vi "Background UI Trigger Timer.vi"(8 "error in (no error)":errorcluster, 10 "Backstage Update Peroid (ms)":i32=-1, 11 "VI Ref (calling VI)":refnum<vi>) -> (0 "error out":errorcluster, 2 "Triggered":bool, 3 "VI Ref (calling VI) (dup)":refnum<vi>)   [LabVIEW 2017]
uses:
  <userlib>/_OpenG.lib/appcontrol/appcontrol.llb/Current VIs Parents Ref__ogtk.vi
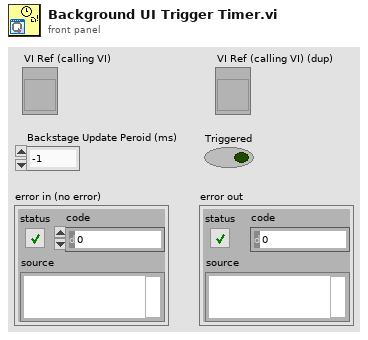
[diagram p1: front panel]
types:
  T1 = enum32{"Invalid", "Standard", "Closed", "Hidden", "Minimized", "Maximized"}
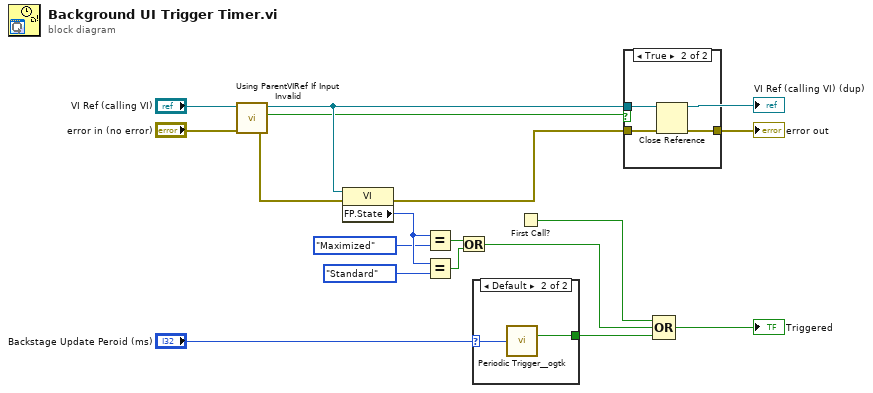
[diagram p0: block diagram]
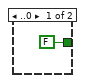
[diagram p2: hidden frame]
diagram:
  n1 = call "Using ParentVIRef If Input Invalid.vi"("VI Ref (calling VI)"="VI Ref (calling VI)") -> ("Using Parent Ref(Need to Destroy)"=w3:bool, "VI Ref"=w4:refnum<vi>)  [unwired: 5 in]
  "VI Ref (calling VI) (dup)" <- w4
  n2 = property on="Property Node" class="VI"(reference=w4, error in="error in (no error)") -> (error out=w16:errorcluster, "FP.State"=w9:T1)  [unwired: 1 out]
  n3 = Equal?(x=w9, y=T1."Maximized") -> (x = y?=w10:bool)
  n4 = Equal?(x=w9, y=T1."Standard") -> (x = y?=w11:bool)
  n5 = Or(x=w10, y=w11) -> (x .or. y?=w12:bool)
  n6 = case shown="Default" "Backstage Update Peroid (ms)" {
    selector: "Backstage Update Peroid (ms)" -> [_ w19]
    tunnel: [FALSE ("time up?") w18] -> w1
    frame ..0 {
    }
    frame Default {
      n7 = call <userlib>:"Periodic Trigger__ogtk.vi"("time (ms)"=w19) -> ("Triggered"=w18:bool)  [unwired: 12 in, 2 out]
    }
  }
  n8 = First Call?() -> (First Call?: T/F=w14:bool)
  n9 = case shown="True" w3 {
    tunnel: w16 -> [w20 w23]
    tunnel: [w20 w22] -> w5
    tunnel: w4 -> [_ w21]
    frame False {
    }
    frame True {
      n10 = Close Reference(reference=w21, error in (no error)=w23) -> (error out=w22:errorcluster)
    }
  }
  "error out" <- w5
  n11 = Compound Arithmetic op=OR(w14, w12, w1) -> (→"Triggered":bool)
